vi "Track Best Ball.vi"(8 "Tracking mode":T4, 9 "Ball Camera Type":T1, 10 "Camera Image":T3, 11 "Ranked Balls":T5(array[cluster]) {"Score" format="%#.1g"}) -> (3 "Ball Track Cluster":T2)   [LabVIEW 2015]
uses:
  Common Code/Tracking Mode.ctl
  <vilib>/vision/Image Controls.llb/IMAQ Image.ctl
  Common Code/Ball Tracking Command Cluster.ctl
  Camera Types.ctl
panel:
  in  "Ball Camera Type 2":T1
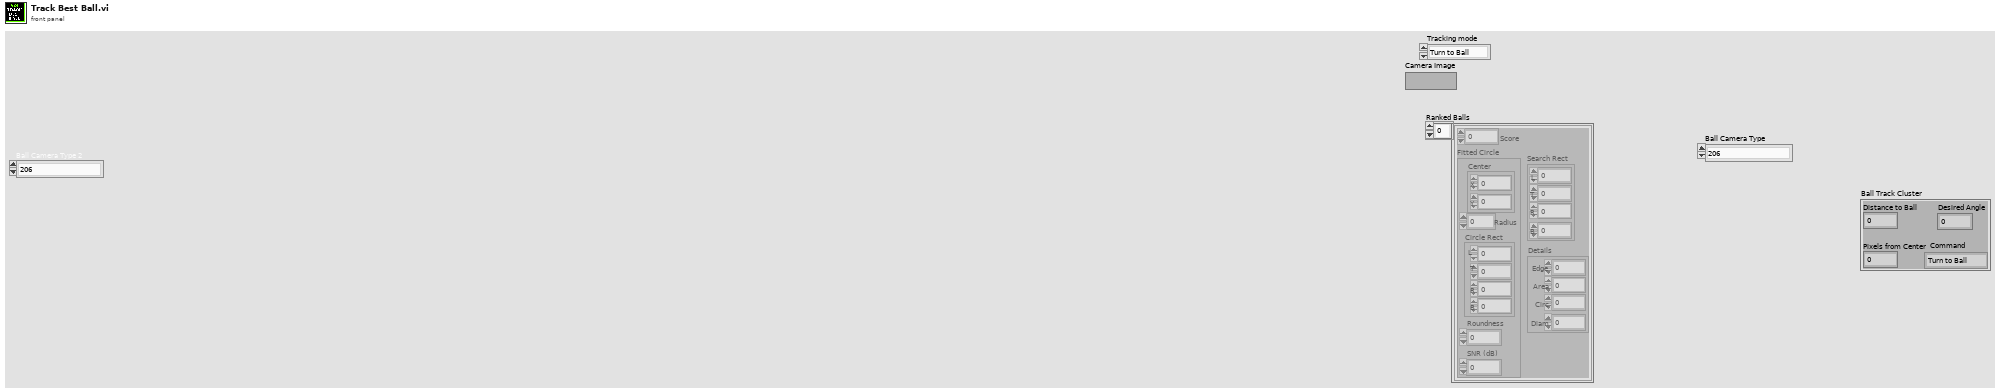
[diagram p1: front panel]
types:
  T1 = typedef "Camera Types.ctl" = enum16{"206", "1011", "1013", "MS HD3000 square", "MS HD3000 640x480"}
  T2 = typedef "Ball Tracking Command Cluster.ctl" = cluster{"Distance to Ball":dbl, "Desired Angle":dbl, "Command":enum16{"Turn to Ball", "Turn to Angle", "Get Distance"}, "Pixels from Center":dbl}
  T3 = typedef "IMAQ Image.ctl" = refnum<image>
  T4 = typedef "Tracking Mode.ctl" = enum16{"Turn to Ball", "Turn to Angle"}
  T5 = cluster{"Score":sgl, "Fitted Circle":cluster{"Center":cluster{"X":sgl, "Y":sgl}, "Radius":dbl, "Circle Rect":cluster{"L":sgl, "T":sgl, "R":sgl, "B":sgl}, "Roundness":dbl, "SNR (dB)":dbl}, "Search Rect":cluster{"L":sgl, "T":sgl, "R":sgl, "B":sgl}, "Details":cluster{"Edge":sgl, "Area":sgl, "Circ":sgl, "Diam":sgl}}[]
  T6 = typedef "Image Type" = u32
  T7 = cluster{"Score":sgl, "Fitted Circle":cluster{"Center":cluster{"X":sgl, "Y":sgl}, "Radius":dbl, "Circle Rect":cluster{"L":sgl, "T":sgl, "R":sgl, "B":sgl}, "Roundness":dbl, "SNR (dB)":dbl}, "Search Rect":cluster{"L":sgl, "T":sgl, "R":sgl, "B":sgl}, "Details":cluster{"Edge":sgl, "Area":sgl, "Circ":sgl, "Diam":sgl}}
  T8 = cluster{"Center":cluster{"X":sgl, "Y":sgl}, "Radius":dbl, "Circle Rect":cluster{"L":sgl, "T":sgl, "R":sgl, "B":sgl}, "Roundness":dbl, "SNR (dB)":dbl}
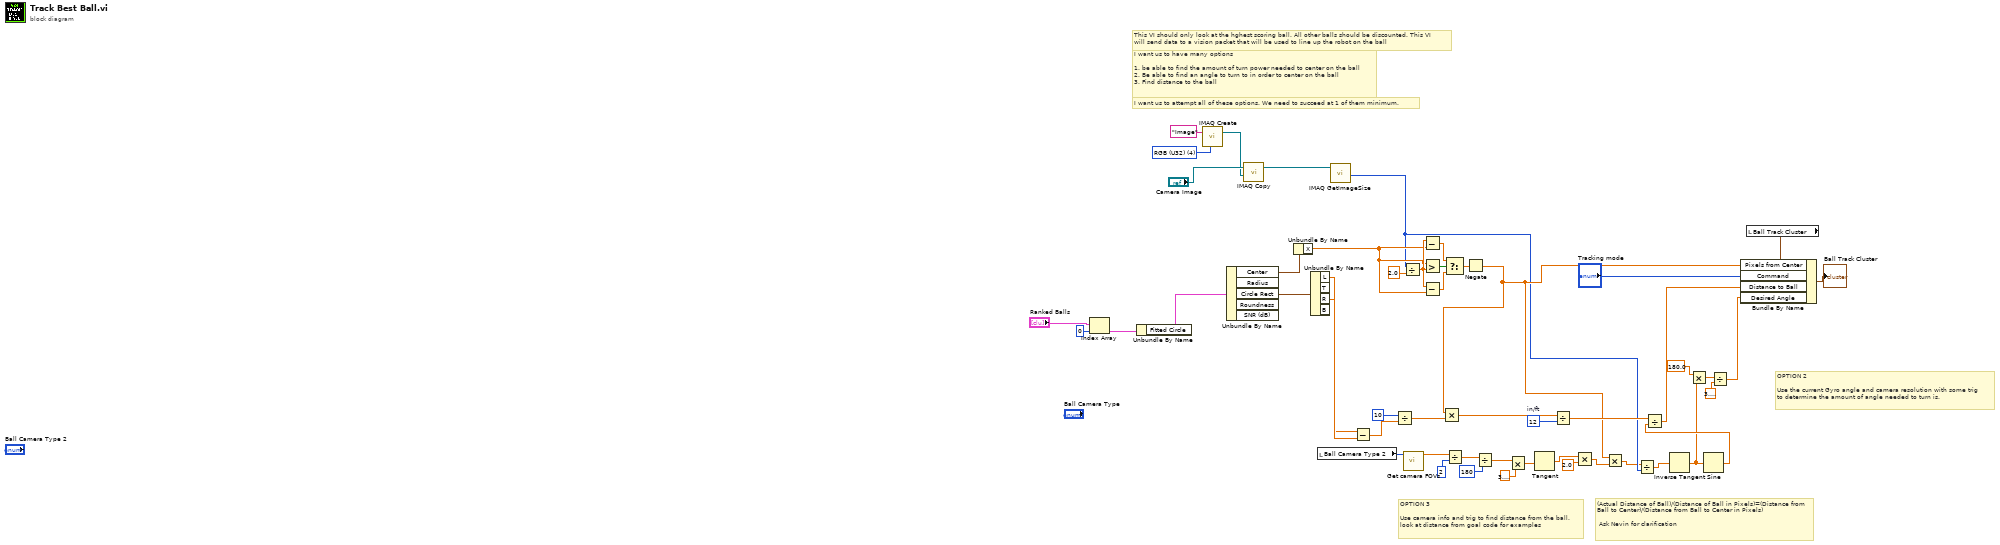
[diagram p0: block diagram]
diagram:
  w32 = 12  # in/ft
  w43 = T6 4 items=["Grayscale (U8)", "Grayscale (I16)", "Grayscale (SGL)", "Complex (CSG)", "RGB (U32)", "HSL (U32)", "RGB (U64)", "Grayscale (U16)"] ("Image Type")
  # "(Actual Distance of Ball)/(Distance of Ball in Pixels)=(Distance from Ball to Center)/(Distance from Ball to Center in Pixels) \n\n Ask Nevin for clarification"
  # "OPTION 3\n\nUse camera info and trig to find distance from the ball.\nlook at distance from goal code for examples"
  # "This VI should only look at the hghest scoring ball. All other balls should be discounted. This VI\nwill send data to a vision packet that will be used to line up the robot on the ball"
  # "I want us to attempt all of these options. We need to succeed at 1 of them minimum."
  # "OPTION 2\n\nUse the current Gyro angle and camera resolution with some trig\nto determine the amount of angle needed to turn is."
  # "I want us to have many options\n\n1. be able to find the amount of turn power needed to center on the ball\n2. Be able to find an angle to turn to in order to center on the ball\n3. Find distance to the ball"
  n1 = Index Array(array="Ranked Balls", index=0) -> (element=w49:T7)
  n2 = Unbundle By Name(w49) -> ("Fitted Circle"=w48:T8)
  n3 = call "IMAQ Create"("Image Name"="Image", "Image Type"=w43) -> ("New Image"=w46:T3)  [unwired: 3 in, 1 out]
  n4 = Unbundle By Name(w48) -> ("Center"=w22:cluster{"X":sgl, "Y":sgl}, "Circle Rect"=w21:cluster{"L":sgl, "T":sgl, "R":sgl, "B":sgl})  [unwired: 3 out]
  n5 = call "IMAQ Copy"("Image Dst"=w46, "Image Src"="Camera Image") -> ("Image Dst Out"=w45:T3)  [unwired: 4 in, 1 out]
  n6 = Unbundle By Name(w22) -> ("X"=w18:sgl)
  n7 = Unbundle By Name(w21) -> ("L"=w20:sgl, "R"=w19:sgl)  [unwired: 2 out]
  n8 = local read "Ball Camera Type 2"() -> (w27:T1)
  n9 = call "IMAQ GetImageSize"("Image"=w45) -> ("X Resolution"=w9:i32)  [unwired: 3 in, 2 out]
  n10 = Subtract(x=w19, y=w20) -> (x-y=w34:sgl)
  n11 = Divide(x=10, y=w34) -> (x/y=w35:sgl)
  n12 = Divide(x=w9, y=2.0) -> (x/y=w41:dbl)
  n13 = call "Get camera FOVs.vi"("Camera Type"=w27) -> ("FOV"=w28:dbl)  [unwired: 9 in, 1 out]
  n14 = Subtract(x=w41, y=w18) -> (x-y=w17:dbl)
  n15 = Greater?(x=w18, y=w41) -> (0:w38:bool)
  n16 = Subtract(x=w41, y=w18) -> (x-y=w40:dbl)
  n17 = Select(t=w17, s=w38, f=w40) -> (s? t:f=w16:dbl)
  n18 = Divide(x=w28, y=2) -> (x/y=w29:dbl)
  n19 = Negate(x=w16) -> (-x=w10:dbl)
  n20 = Multiply(x=w10, y=w35) -> (x*y=w36:dbl)
  n21 = Divide(x=w29, y=180) -> (x/y=w30:dbl)
  n22 = Multiply(x=w30, y=3.141592653589793) -> (x*y=w31:dbl)
  n23 = Tangent(1:w31) -> (0:w13:dbl)
  n24 = Divide(x=w36, y=w32) -> (x/y=w37:dbl)
  n25 = Multiply(x=w13, y=2.0) -> (x*y=w11:dbl)
  n26 = Multiply(x=w10, y=w11) -> (x*y=w8:dbl)
  n27 = Divide(x=w8, y=w9) -> (x/y=w7:dbl)
  n28 = Inverse Tangent(1:w7) -> (0:w4:dbl)
  n29 = Multiply(x=180.0 ("y"), y=w4) -> (x*y=w3:dbl)
  n30 = Sine(x=w4) -> (sin(x)=w6:dbl)
  n31 = Divide(x=w37, y=w6) -> (x/y=w14:dbl)
  n32 = Divide(x=w3, y=3.141592653589793) -> (x/y=w1:dbl)
  n33 = local read "Ball Track Cluster"() -> (w42:T2)
  n34 = Bundle By Name(cluster=w42, "Pixels from Center"=w10, "Command"="Tracking mode", "Distance to Ball"=w14, "Desired Angle"=w1) -> (→"Ball Track Cluster":T2)
